vi "DAQmx Switch Name.vi"(1 "DAQmx Switch Name":tag) -> (0 "DAQmx Switch Name Out":tag)   [LabVIEW 2011]
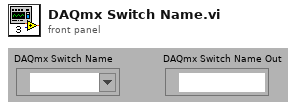
[diagram p1: front panel]
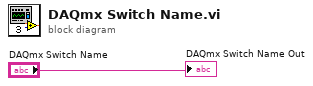
[diagram p0: block diagram]
diagram:
  "DAQmx Switch Name Out" <- "DAQmx Switch Name"
